vi "MES_Get StationData.vi"(0 "LineNum":string, 5 "StationName":string, 11 "error in (no error)":errorcluster, 12 "Alarm":bool=TRUE) -> (4 "Value":T1, 10 "Total Results":string[][](table), 13 "Table Control":string[][](array[string]), 14 "PLC DB DBB1List":string[](array[string]), 15 "error out":errorcluster)   [LabVIEW 2017, in "SQLite.lvclass"]
doc: "获取工位的使用的DB，结果DB，交互信号DB，报警DB，设备状态-结果分类-Andon报警DB、\n#2020-5-23 10:10:02\n蒋松\njiangsong@outlook.com"
uses:
  SQLite.lvclass
  Control/Station value Type.ctl
  SQLiteFileName.ctl
  TabelFullName.ctl
  <userlib>/LabSQL/LabSQL.lvlib
  <userlib>/sushu/sushu.lvlib
panel:
  in  "String":string
  out "number (0 to 1)":dbl
  out "Select SQL CMD":string
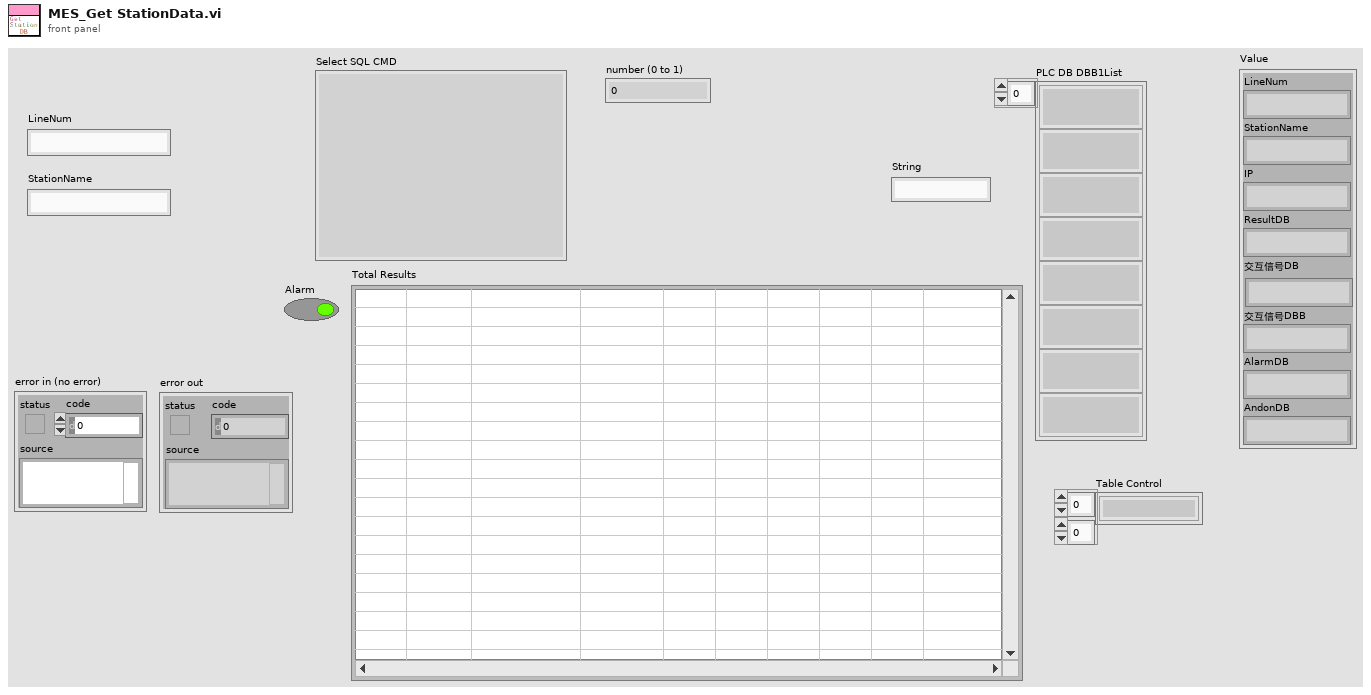
[diagram p1: front panel]
types:
  T1 = typedef "SQLite.lvclass/Station value Type.ctl" = cluster{"LineNum":string, "StationName":string, "IP":string, "ResultDB":string, "交互信号DB":string, "交互信号DBB":string, "AlarmDB":string, "AndonDB":string}
  T2 = enum16{"Initialize", "Read", "Write", "UnInitialize"}
  T3 = typedef "SQLite.lvclass/TabelFullName.ctl" = string
  T4 = typedef "SQLite.lvclass/SQLiteFileName.ctl" = string
  T5 = cluster{"Current VI Reference":refnum<vi>, "Close Panel on Exit?":bool}
  T6 = cluster{"Core":cluster{"Current VI Reference":refnum<vi>, "Close Panel on Exit?":bool}, "VI Name":string}
  T7 = enum16{"Other", "SQL2008", "SQLite", "Access", "MySQL"}
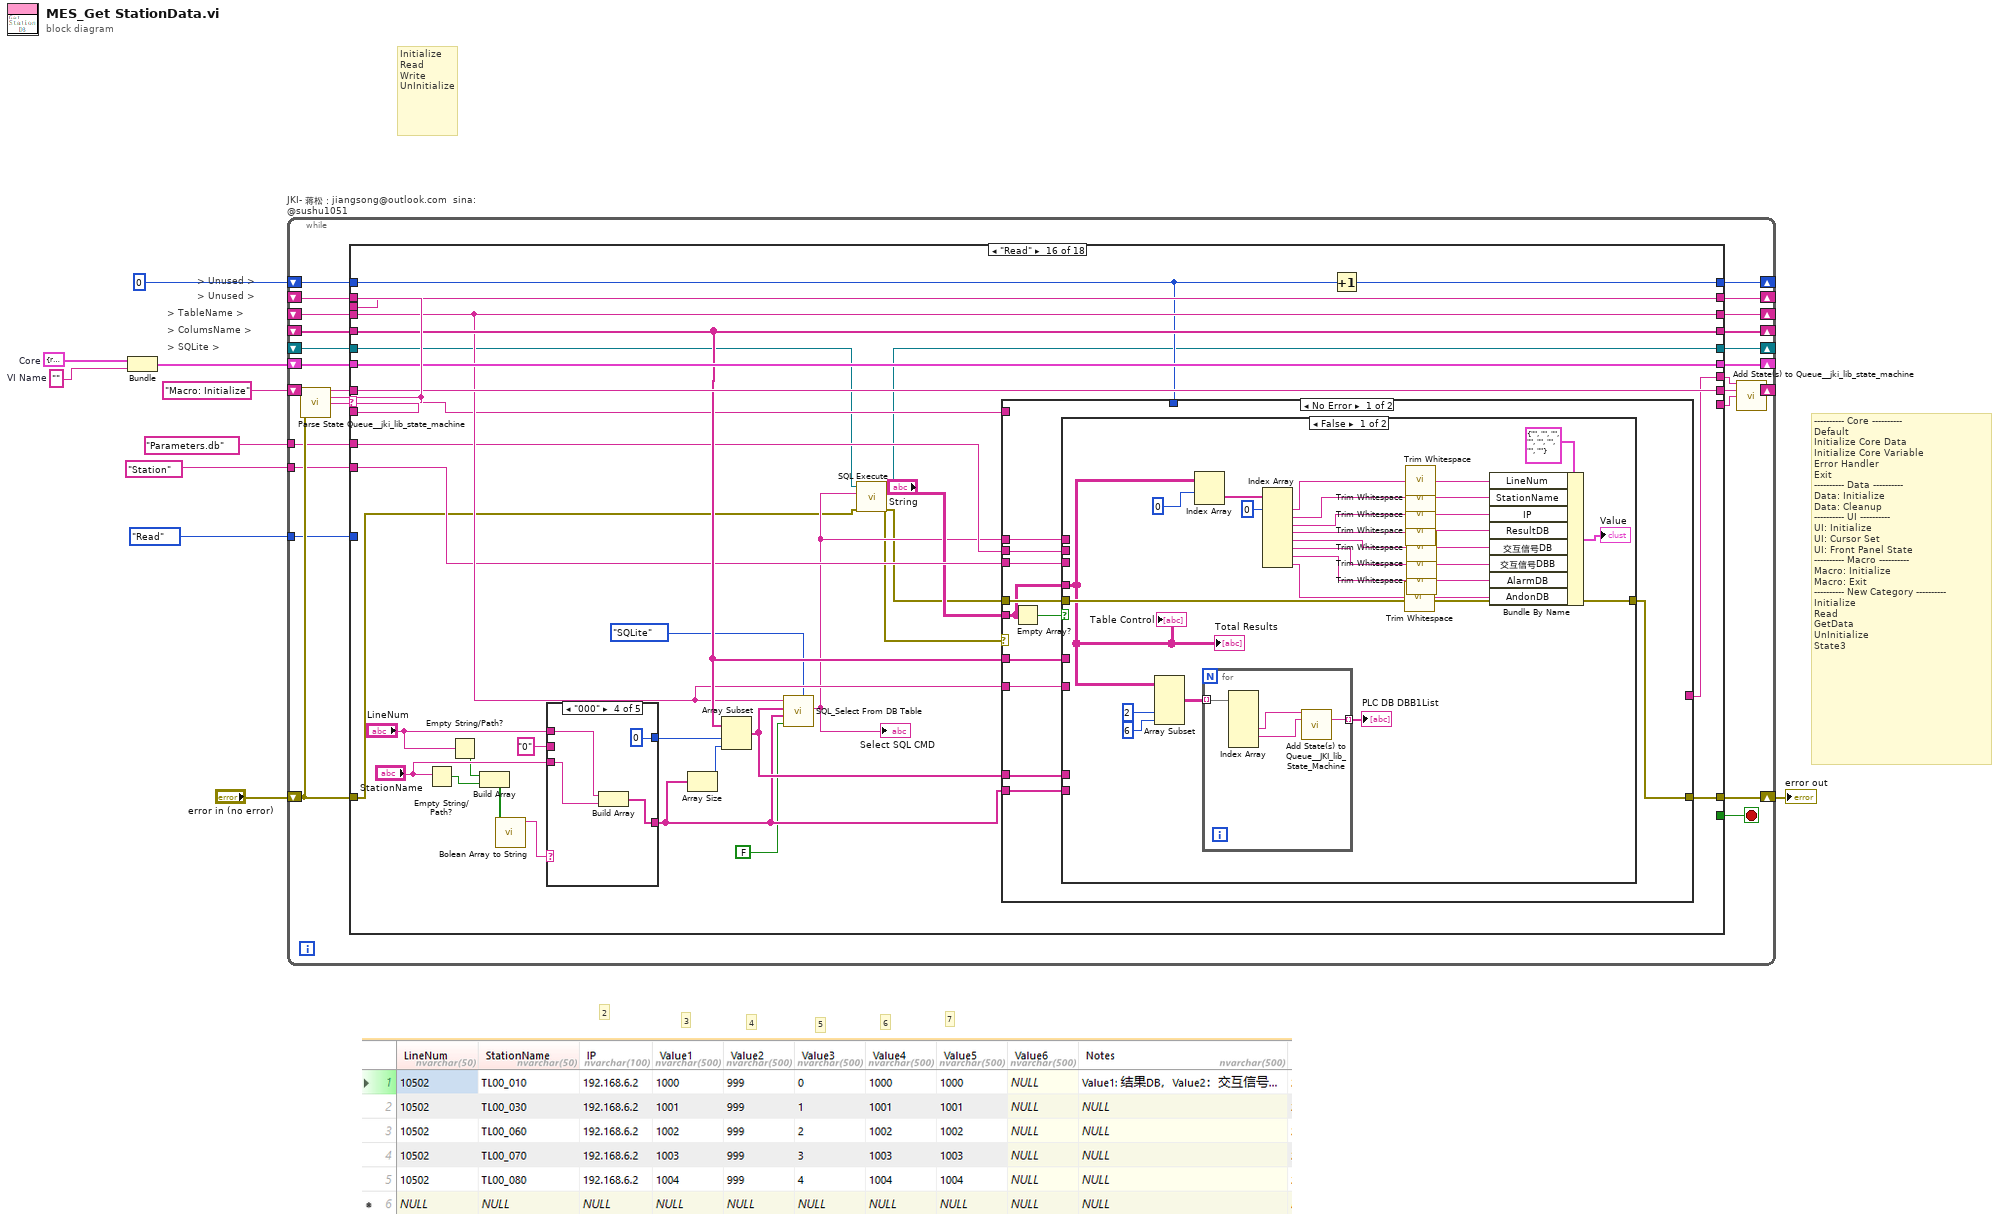
[diagram p0: block diagram]
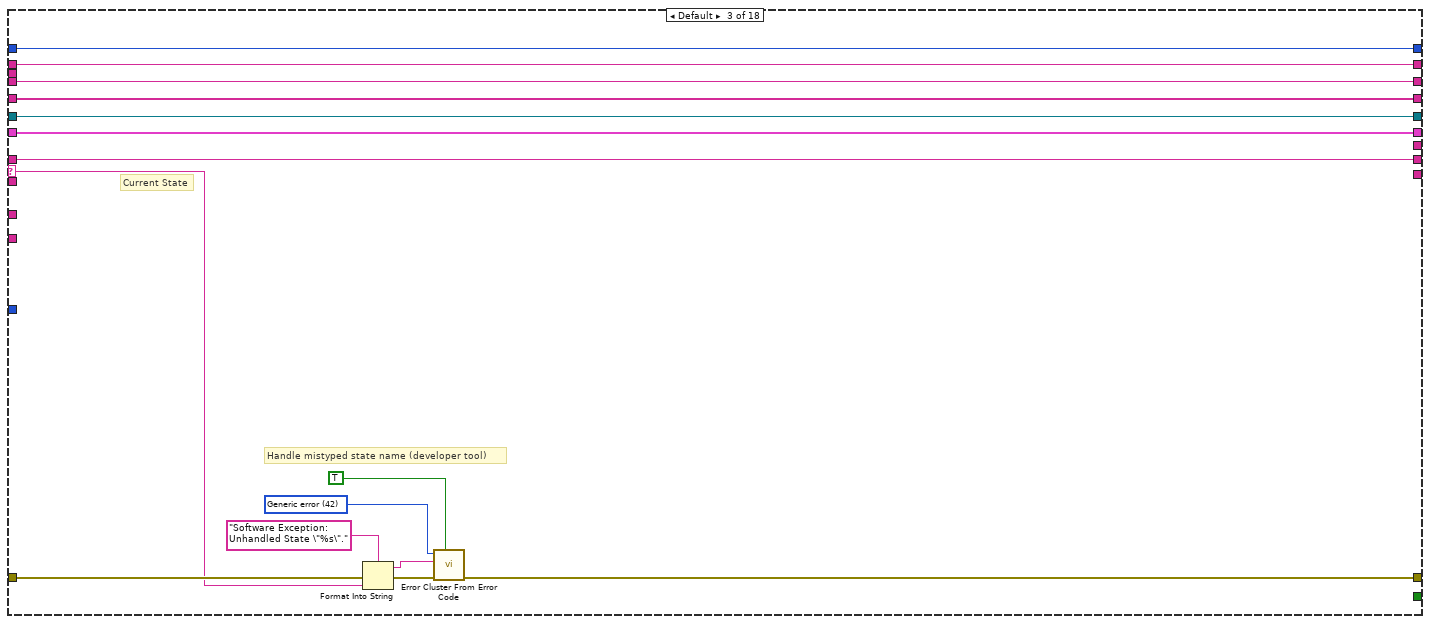
[diagram p4: hidden frame]
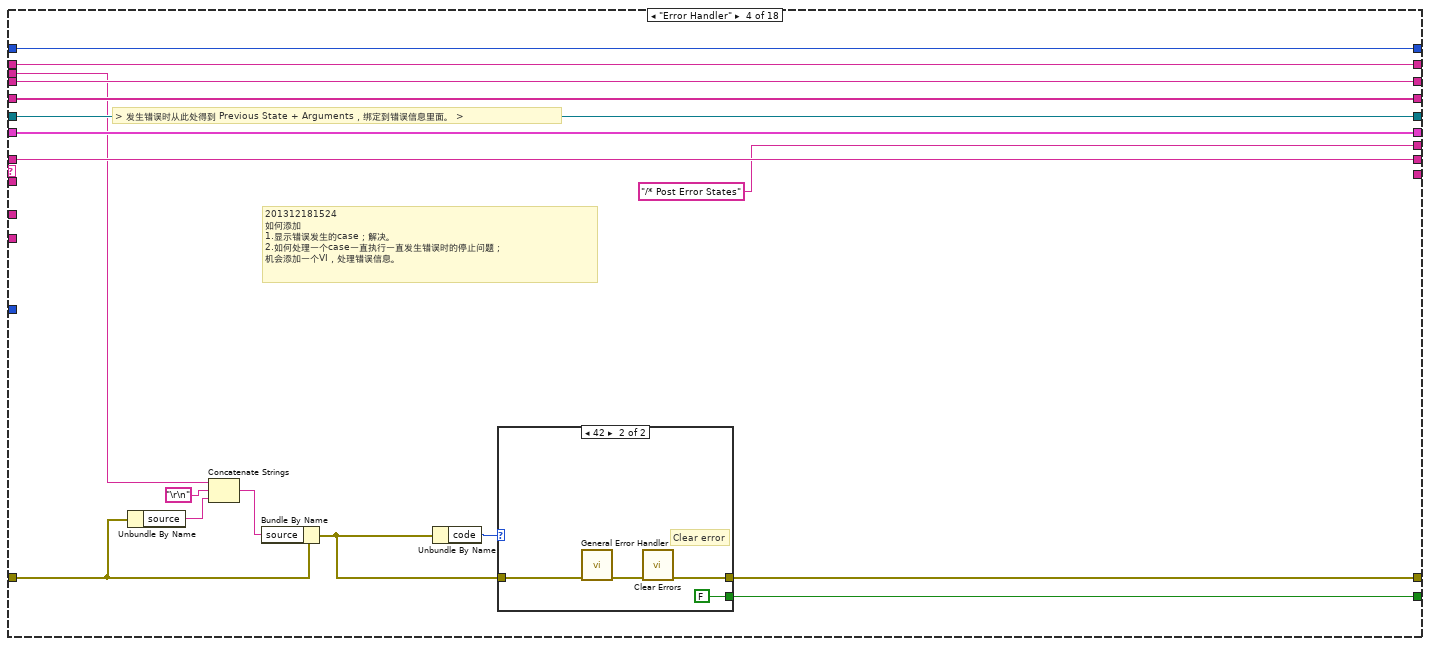
[diagram p5: hidden frame]
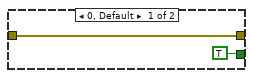
[diagram p6: hidden frame]
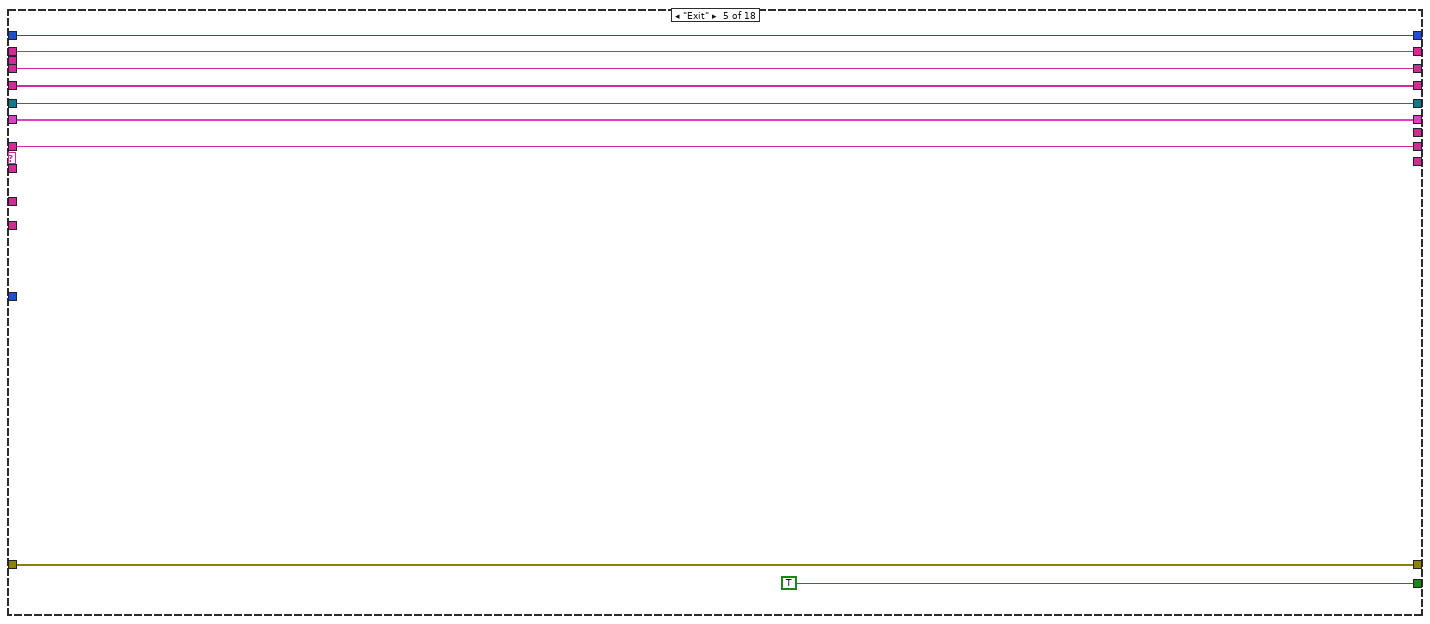
[diagram p7: hidden frame]
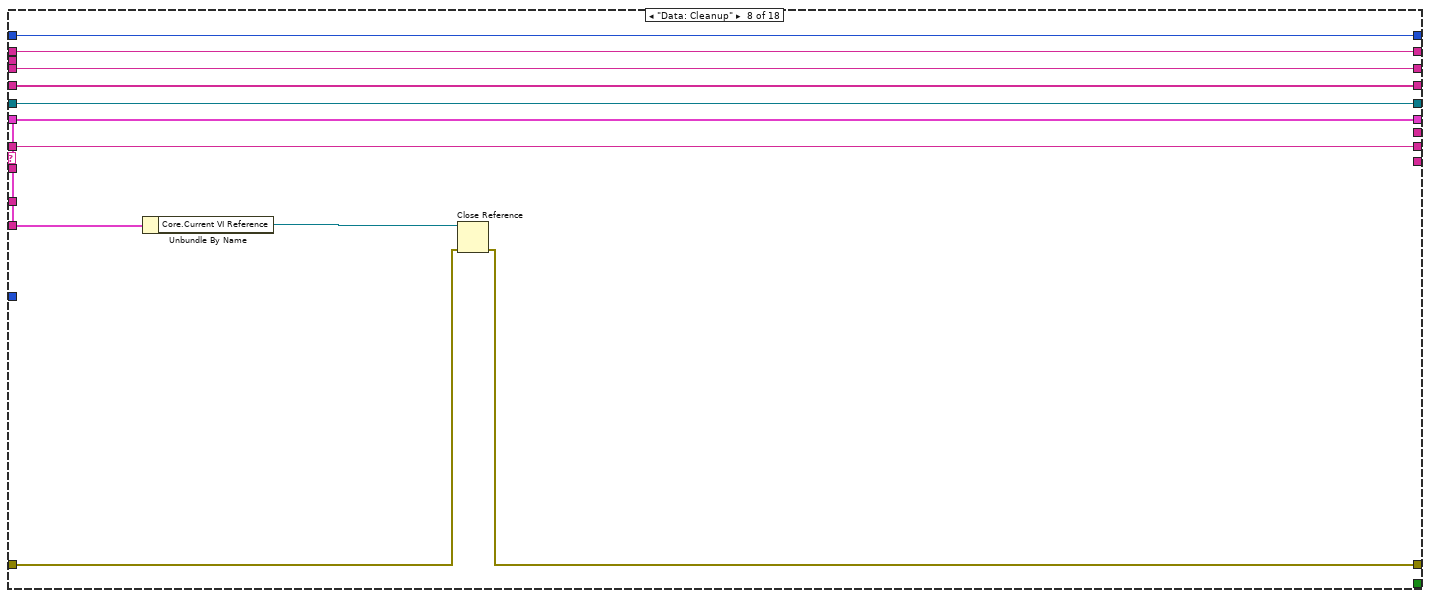
[diagram p10: hidden frame]
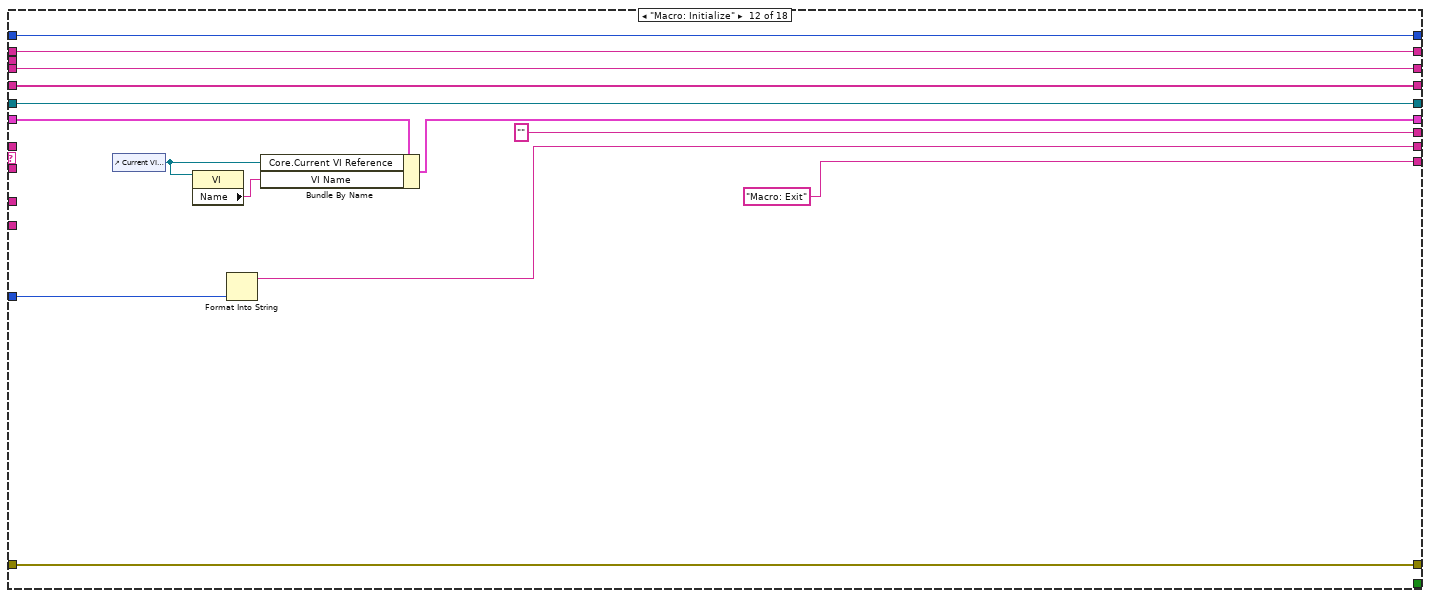
[diagram p14: hidden frame]
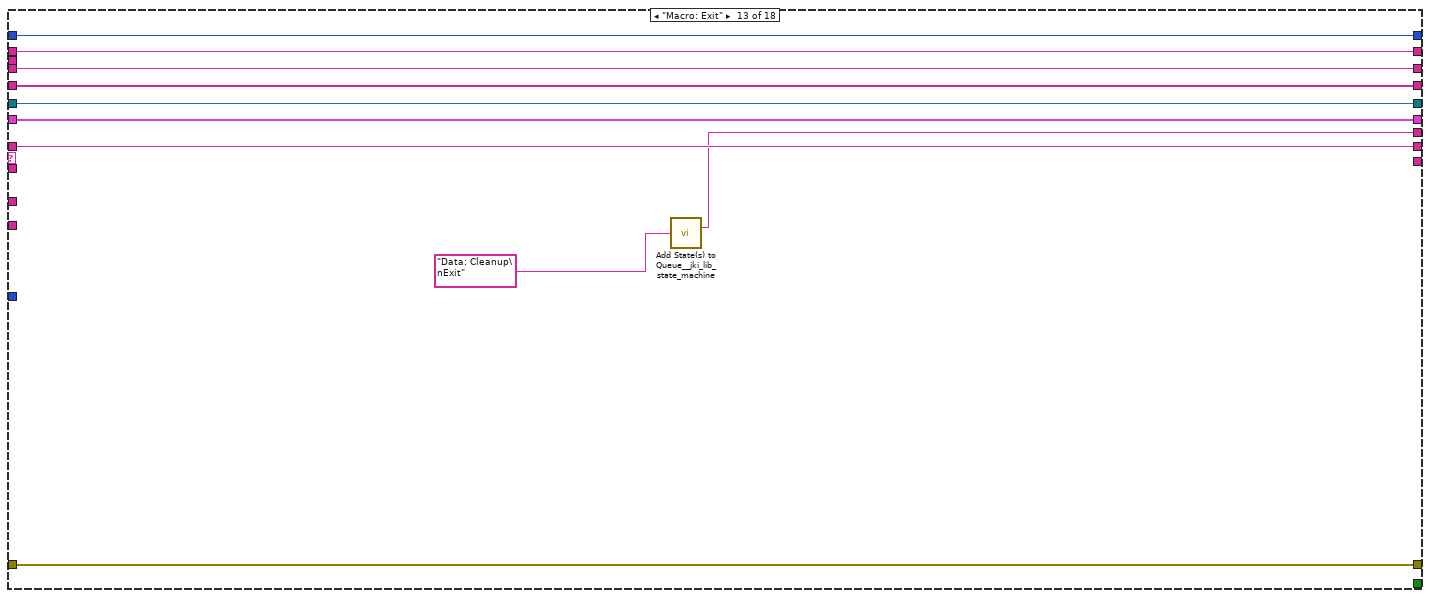
[diagram p15: hidden frame]
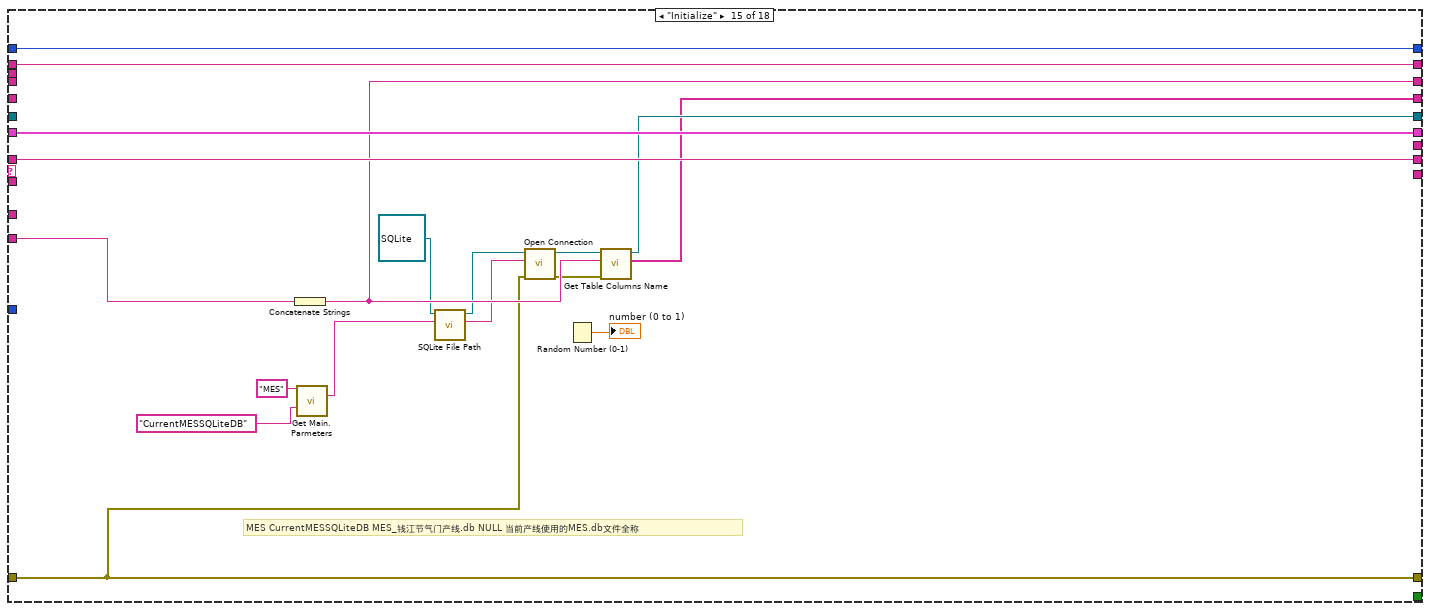
[diagram p17: hidden frame]
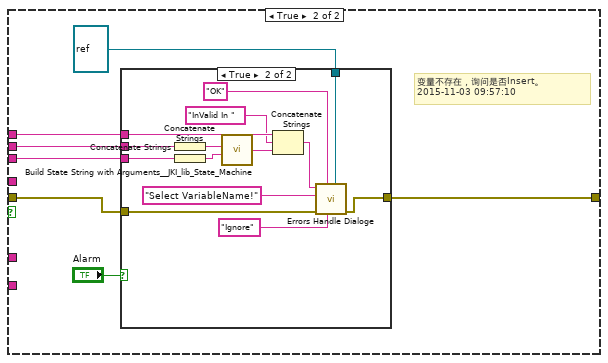
[diagram p18: hidden frame]
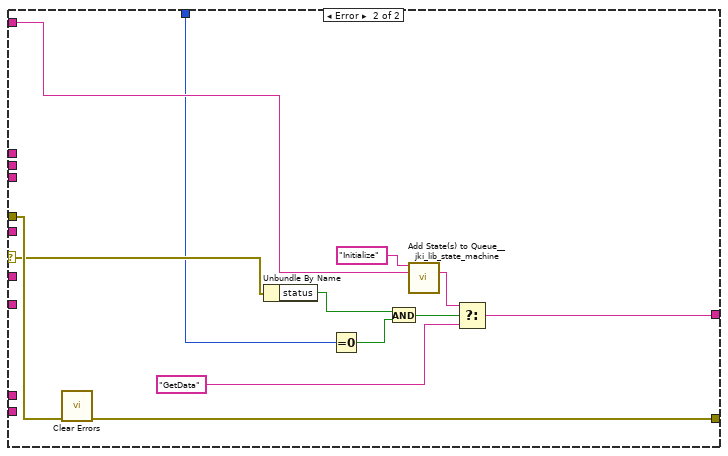
[diagram p20: hidden frame]
diagram:
  w10 = ""  # VI Name
  w9 = T5 {"Current VI Reference"=refnum, "Close Panel on Exit?"=FALSE}  # Core
  # "7"
  # "2"
  # "6"
  # "5"
  # "4"
  # "3"
  # "Initialize\nRead\nWrite\nUnInitialize"
  # "> Unused >"
  # "> SQLite >"
  # "> ColumsName >"
  # "> TableName >"
  # "> Unused >"
  # "---------- Core ----------\nDefault\nInitialize Core Data\nInitialize Core Variable\nError Handler\nExit\n---------- Data ----------\nData: Initialize\nData: Cleanup\n---------- UI ----------\nUI: Initialize\nUI: Cursor Set\nUI: Front Panel State\n---------- Macro ----------\nMacro: Initialize\nMacro: Exit\n---------- New Category ----------\nInitialize\nRead\nGetData\nUnInitialize\nState3"
  n1 = Bundle("Core"=w9, "VI Name"=w10) -> (w8:T6)  [unwired: 1 in]
  n2 = while "JKI- 蒋松：jiangsong@outlook.com  sina: @sushu1051" {
    shift-right: [w34] -> w3
    shift-left: "error in (no error)" -> [w32]
    shift-right: [w22] -> _
    shift-left: "Macro: Initialize" -> [w23]
    shift-right: [w29] -> _
    shift-left: _ -> [w31]
    shift-right: [w30] -> _
    shift-left: _ -> [w11]
    shift-right: [w24] -> _
    shift-left: w8 -> [w27]
    shift-right: [w25] -> _
    shift-left: _ -> [w18]
    shift-right: [w26] -> _
    shift-left: _ -> [w28]
    shift-right: [w17] -> _
    shift-left: 0 -> [w16]
    tunnel: T2."Read" ("CMD") -> [w15]
    tunnel: T4 "Parameters.db" ("SQLiteFileName") -> [w14]
    tunnel: T3 "Station" ("TabelFullName") -> [w13]
    stop <- w33 stop-if-true
    n3 = call <vilib>:"Parse State Queue__jki_lib_state_machine.vi"("State Queue"=w23, "Error In (no error)"=w32) -> ("Remaining States"=w36:string, "Current State"=w12:string, "Arguments"=w35:string)  [unwired: 10 in, 1 out]
    n4 = case shown="\"Read\"" w12 {
      selector: w12 -> [_ _ w55 _ _ _ _ _ _ _ _ _ _ _ _ w217 _ _]
      tunnel: w36 -> [w44 w46 w54 w76 w92 w101 w110 w117 w127 w135 w143 _ w166 w175 w199 w230 w331 w341]
      tunnel: w35 -> [_ _ _ _ _ _ _ _ _ _ _ _ _ _ _ _ _ _]
      tunnel: [w43 w52 w56 w70 w94 w103 w112 w119 w129 w137 w145 w160 w170 w178 w189 w218 w324 w332] -> w34
      tunnel: w32 -> [w43 w52 w57 w80 w94 w103 w112 w120 w129 w137 w145 w160 w170 w178 w189 w210 w324 w333]
      tunnel: [w44 w46 w54 w76 w92 w101 w110 w117 w127 w135 w143 w151 w166 w175 w199 w230 w331 w341] -> w21
      tunnel: [_ _ _ w69 TRUE _ _ _ _ _ _ _ _ _ _ _ _ _] -> w33
      tunnel: w12 -> [w42 w51 w67 w84 w99 w107 w115 w125 w133 w141 w149 w163 w173 w181 w198 w219 w325 w340]
      tunnel: w31 -> [w41 w50 w66 w83 w98 w106 w114 w124 w132 w140 w148 w162 w172 w180 _ w222 w330 w339]
      tunnel: [w42 w51 w67 w84 w99 w107 w115 w125 w133 w141 w149 w163 w173 w181 w198 w219 w325 w340] -> w30
      tunnel: [w41 w50 w66 w83 w98 w106 w114 w124 w132 w140 w148 w162 w172 w180 w191 w222 w330 w339] -> w29
      tunnel: w28 -> [w40 w49 w65 w82 w97 w105 w113 w123 w131 w139 w147 w161 w171 w179 _ w223 w329 w338]
      tunnel: w18 -> [w38 w47 w64 w74 w93 w102 w111 w118 w128 w136 w144 w159 w167 w176 _ w214 w328 w335]
      tunnel: w27 -> [w39 w48 w63 w81 w96 w104 w108 w121 w130 w138 w146 w153 w168 w177 w197 w229 w327 w337]
      tunnel: [w40 w49 w65 w82 w97 w105 w113 w123 w131 w139 w147 w161 w171 w179 w192 w223 w329 w338] -> w26
      tunnel: [w38 w47 w64 w74 w93 w102 w111 w118 w128 w136 w144 w159 w167 w176 w193 w212 w328 w334] -> w25
      tunnel: [w39 w48 w63 w81 w96 w104 w108 w121 w130 w138 w146 w152 w168 w177 w197 w229 w327 w337] -> w24
      tunnel: [_ _ _ "/* Post Error States" _ _ _ _ _ _ _ "" w165 _ _ w216 _ _] -> w20
      tunnel: [_ _ _ _ _ _ _ _ _ _ _ "Macro: Exit" _ _ _ _ _ _] -> w19
      tunnel: w16 -> [w37 w45 w53 w73 w91 w100 w109 w116 w126 w134 w142 w158 w164 w174 w196 w215 w326 w336]
      tunnel: [w37 w45 w53 w73 w91 w100 w109 w116 w126 w134 w142 w158 w164 w174 w196 w228 w326 w336] -> w17
      tunnel: w15 -> [_ _ _ _ _ _ _ _ _ _ _ w150 _ _ _ _ _ _]
      tunnel: w14 -> [_ _ _ _ _ _ _ _ _ _ _ _ _ _ _ w220 _ _]
      tunnel: w13 -> [_ _ _ _ _ _ _ _ _ _ _ _ _ _ w194 w221 _ _]
      tunnel: w11 -> [_ _ _ w68 _ _ _ _ _ _ _ _ _ _ _ _ _ _]
      frame "Idle" {
      }
      frame "---------- Core ----------" {
      }
      frame Default {
        w59 = 42 items=["No error", "Argument error", "Memory is full", "Out of zone", "End of file", "File already open", "Generic file I/O error", "File not found", "File permission error", "Disk is full", "Duplicate path", "Too many files open", "System feature not enabled", "Resource file not found", "Cannot add resource", "Resource not found", "Image not found", "Image memory error", "Pen does not exist", "Config type invalid", "Config token not found", "Config parse error", "Config memory error", "Bad external code format", "Bad external code offset", "External code not present", "Null window", "Destroy window error", "Null menu", "Print aborted", "Bad print record", "Print driver error", "Windows error during printing", "Memory error during printing", "Print dialog error", "Generic print error", "Invalid device refnum", "Device not found", "Device parameter error", "Device unit error", "Cannot open device", "Device call aborted", "Generic error", "Cancelled by user", "Object ID too low", "Object ID too high", "Object not in heap", "Unknown heap", "Unknown object (invalid DefProc)", "Unknown object (DefProc not in table)", "Message out of range", "Invalid (null) method", "Unknown message", "Manager call not supported", "Bad address", "Network operation in progress", "Network operation timed out", "Connection is busy", "Network attribute not supported", "Network error", "Address in use", "System out of memory", "Connection aborted", "Connection refused", "Not connected", "Already connected", "Connection closed", "Initialization error (interapplication manager)", "Bad occurrence", "Wait on unbound occurrence handler", "Occurrence queue overflow", "Datalog type conflict", "Unused", "Unrecognized type (interapplication manager)", "Memory corrupt", "Failed to make temporary DLL", "Old CIN version", "Drag socket not found", "Failed to load drop-object", "Failed to register OLE object", "Failed to release OLE object", "Format specifier type mismatch", "Unknown format specifier", "Too few format specifiers", "Too many format specifiers", "Scan failed", "Newer CIN version", "Error converting to variant", "Runtime menu error", "Password tampered", "Variant attribute not found", "Incompatible variant data type", "Event data is not available", "Event Store is not present", "Occurrence is not found", "Event Queue is not created", "Event info is not available", "Refnum passed is NULL", "Error retrieving Class GUID", "Error retrieving CoClass GUID", "Error retrieving TypeLib GUID.", "Bad built application magic bytes.", "Specific driver is different from the specific driver associated with the Logical Name.", "There is no session opened to the class driver.", "Max Error", "MAX - Error with config objects", "MAX - Error loading configuration", "MAX - Group not supported"]
        # "Current State"
        # "Handle mistyped state name (developer tool)"
        n5 = Format Into String(format string="Software Exception: Unhandled State \"%s\"." ("message"), error in=w57, w55) -> (resulting string=w60:string, error out=w61:errorcluster)  [unwired: 1 in]
        n6 = call <vilib>:"Error Cluster From Error Code.vi"("show call chain? (False)"=TRUE, "error in (no error)"=w61, "error message (\"\")"=w60, "error code (0)"=w59) -> ("error out"=w56:errorcluster)  [unwired: 5 in]
      }
      frame "Error Handler" {
        # "> 发生错误时从此处得到 Previous State + Arguments，绑定到错误信息里面。 >"
        # "201312181524\n如何添加\n1.显示错误发生的case；解决。\n2.如何处理一个case一直执行一直发生错误时的停止问题；\n机会添加一个VI，处理错误信息。"
        # "Clear error"
        n7 = Unbundle By Name(w80) -> ("source"=w78:string)
        n8 = Concatenate Strings(w68, "\r\n", w78) -> (w77:string)
        n9 = Bundle By Name(cluster=w80, "source"=w77) -> (w71:errorcluster)
        n10 = Unbundle By Name(w71) -> ("code"=w72:i32)
        n11 = case shown="42" w72 {
          tunnel: [TRUE FALSE] -> w69
          tunnel: w71 -> [w86 w89]
          tunnel: [w86 w87] -> w70
          frame 0, Default {
          }
          frame 42 {
            n12 = call <vilib>:"General Error Handler.vi"("error in (no error)"=w89) -> ("error out"=w88:errorcluster)  [unwired: 10 in, 4 out]
            n13 = call <vilib>:"Clear Errors.vi"("error in (no error)"=w88) -> ("error out"=w87:errorcluster)  [unwired: 5 in, 1 out]
          }
        }
      }
      frame "Exit" {
      }
      frame "---------- Data ----------" {
      }
      frame "Data: Initialize" {
      }
      frame "Data: Cleanup" {
        n14 = Unbundle By Name(w121) -> ("Core.Current VI Reference"=w122:refnum<vi>)
        n15 = Close Reference(reference=w122, error in (no error)=w120) -> (error out=w119:errorcluster)
      }
      frame "---------- UI ----------" {
      }
      frame "UI: Initialize" {
      }
      frame "---------- Macro ----------" {
      }
      frame "Macro: Initialize" {
        n16 = control-ref of="Current VI Reference"() -> (w154:refnum<vi>)
        n17 = property class="VI"(reference=w154) -> ("Name"=w155:string)  [unwired: 1 in, 2 out]
        n18 = Format Into String(w150) -> (resulting string=w151:string)  [unwired: 3 in, 1 out]
        n19 = Bundle By Name(cluster=w153, "Core.Current VI Reference"=w154, "VI Name"=w155) -> (w152:T6)
      }
      frame "Macro: Exit" {
        n20 = call <vilib>:"Add State(s) to Queue__jki_lib_state_machine.vi"("State(s) at Back (\"\")"="Data: Cleanup\nExit") -> ("States Out"=w165:string)  [unwired: 14 in]
      }
      frame "---------- New Category ----------" {
      }
      frame "Initialize" {
        # "MES\tCurrentMESSQLiteDB\tMES_钱江节气门产线.db\tNULL\t当前产线使用的MES.db文件全称"
        n21 = Concatenate Strings(w194) -> (w191:string)
        n22 = call "Get Main.Parmeters.vi"("Main"="MES", "VariableName"="CurrentMESSQLiteDB" ("Main")) -> ("Value"=w182:string)  [unwired: 6 in, 7 out]
        n23 = call "SQLite File Path.vi"("SQLiteFileName"=w182, "SQLite in"=refnum<class "SQLite.lvclass"> refnum ("SQLite.lvclass")) -> ("string"=w188:string, "SQLite out"=w186:refnum<class "SQLite.lvclass">)  [unwired: 7 in, 1 out]
        n24 = call-dynamic "Open Connection.vi"("error in (no error)"=w189, "ConnectionString"=w188, "HostDB in"=w186) -> ("error out"=w190:errorcluster, "HostDB out"=w195:refnum<class "SQLite.lvclass">)  [unwired: 7 in]
        n25 = Random Number (0-1)() -> (number: 0 to 1=→"number (0 to 1)":dbl)
        n26 = call-dynamic "Get Table Columns Name.vi"("error in (no error)"=w190, "TableName"=w191, "HostDB in"=w195) -> ("Table_ColunmsList"=w192:string[], "HostDB out"=w193:refnum<class "SQLite.lvclass">)  [unwired: 4 in, 3 out]
      }
      frame "Read" {
        n27 = Empty String/Path?(string/path="StationName") -> (empty?=w207:bool)
        n28 = Empty String/Path?(string/path="LineNum") -> (empty?=w202:bool)
        n29 = Build Array(w202, w207) -> (w206:bool[])
        n30 = call <userlib>:"Bolean Array to String.vi"("Bolean Array"=w206) -> ("Bolean String"=w205:string)  [unwired: 10 in]
        n31 = case shown="\"000\"" w205 {
          tunnel: [w309 w312 w315 w319 w323] -> w226
          tunnel: "StationName" -> [w307 _ _ w316 w322]
          tunnel: [1 ("index") 2 ("index") 0 ("index") 0 ("index") 0 ("index")] -> w203
          tunnel: "LineNum" -> [_ _ w313 w317 w320]
          tunnel: "0" ("element") -> [_ _ _ _ _]
          frame "10" {
            n32 = Build Array(w307) -> (w309:string[])
          }
          frame "11" {
            n33 = Build Array("" ("element")) -> (w312:string[])
          }
          frame "01" {
            n34 = Build Array(w313) -> (w315:string[])
          }
          frame "000" {
            n35 = Build Array(w317, w316) -> (w319:string[])
          }
          frame "False", Default {
            n36 = Build Array(w320, w322) -> (w323:string[])
          }
        }
        n37 = Array Size(array=w226) -> (size(s)=w225:i32)
        n38 = Array Subset(array=w223, index=w203, length=w225) -> (w227:string[])
        n39 = call <userlib>:"SQL_Select From DB Table.vi"("DB Type"=T7."SQLite", "Check ASCII?"=FALSE, "ColumnsValue"=w226, "ColumnsNameList"=w227, "TableName"=w222) -> ("Select SQL CMD"=w211:string)  [unwired: 6 in]
        "Select SQL CMD" <- w211
        n40 = call-dynamic "SQL Execute.vi"("error in (no error)"=w210, "Command Text"=w211, "HostDB in"=w214) -> ("error out"=w209:errorcluster, "Table Control"=w213:string[][], "HostDB out"=w212:refnum<class "SQLite.lvclass">)  [unwired: 4 in, 2 out]
        n41 = case shown="No Error" w209 {
          selector: w209 -> [_ w299]
          tunnel: w227 -> [w241 _]
          tunnel: w209 -> [w240 w306]
          tunnel: w211 -> [w238 _]
          tunnel: w213 -> [w237 _]
          tunnel: w226 -> [w236 _]
          tunnel: w223 -> [w235 _]
          tunnel: w222 -> [w234 _]
          tunnel: w221 -> [w233 _]
          tunnel: w220 -> [w232 _]
          tunnel: [w231 w305] -> w218
          tunnel: w217 -> [_ w298]
          tunnel: [_ w297] -> w216
          tunnel: w215 -> [_ w296]
          frame No Error {
            n42 = Empty Array?(array=w237) -> (empty?=w239:bool)
            n43 = case shown="False" w239 {
              tunnel: [w268 w278] -> w231
              tunnel: w235 -> [_ _]
              tunnel: w234 -> [_ _]
              tunnel: w236 -> [_ _]
              tunnel: w241 -> [_ _]
              tunnel: w240 -> [w268 w279]
              tunnel: w238 -> [_ w275]
              tunnel: w232 -> [_ w277]
              tunnel: w233 -> [_ w276]
              tunnel: w237 -> [w254 _]
              frame False {
                n44 = Array Subset(array=w254, index (col)=2 ("index"), length (col)=6 ("length")) -> (w259:string[][])  [unwired: 2 in]
                n45 = Index Array(array=w254, index (row)=0) -> (element=w266:string[])  [unwired: 1 in]
                n46 = for {
                  tunnel: w259 -> [w272] mode=indexing
                  tunnel: [w271] -> w258 mode=indexing
                  n47 = Index Array(array=w272) -> (element #3=w270:string, element #4=w269:string)  [unwired: 5 in, 3 out]
                  n48 = call <vilib>:"Add State(s) to Queue__JKI_lib_State_Machine.vi"("State(s) in Front (\"\")"=w270, "State(s) in (\"\")"=w269) -> ("States Out"=w271:string)  [unwired: 13 in]
                }
                "PLC DB DBB1List" <- w258
                n49 = Index Array(array=w266, index #1=0 ("index")) -> (element #1=w265:string, element #2=w264:string, element #3=w263:string, element #4=w262:string, element #5=w247:string, element #6=w246:string, element #7=w245:string, element #8=w244:string)  [unwired: 7 in]
                n50 = call <vilib>:"Trim Whitespace.vi"("string"=w244) -> ("trimmed string"=w243:string)  [unwired: 1 in]
                n51 = call <vilib>:"Trim Whitespace.vi"("string"=w265) -> ("trimmed string"=w257:string)  [unwired: 1 in]
                n52 = call <vilib>:"Trim Whitespace.vi"("string"=w264) -> ("trimmed string"=w256:string)  [unwired: 1 in]
                n53 = call <vilib>:"Trim Whitespace.vi"("string"=w263) -> ("trimmed string"=w255:string)  [unwired: 1 in]
                n54 = call <vilib>:"Trim Whitespace.vi"("string"=w262) -> ("trimmed string"=w250:string)  [unwired: 1 in]
                n55 = call <vilib>:"Trim Whitespace.vi"("string"=w247) -> ("trimmed string"=w249:string)  [unwired: 1 in]
                n56 = call <vilib>:"Trim Whitespace.vi"("string"=w246) -> ("trimmed string"=w248:string)  [unwired: 1 in]
                n57 = call <vilib>:"Trim Whitespace.vi"("string"=w245) -> ("trimmed string"=w242:string)  [unwired: 1 in]
                n58 = Bundle By Name(cluster=T1 {"LineNum"="", "StationName"="", "IP"="", "ResultDB"="", "交互信号DB"="", "交互信号DBB"="", "AlarmDB"="", "AndonDB"=""} ("Value"), "LineNum"=w257, "StationName"=w256, "IP"=w255, "ResultDB"=w250, "交互信号DB"=w249, "交互信号DBB"=w248, "AlarmDB"=w242, "AndonDB"=w243) -> (→"Value":T1)
                "Total Results" <- w254
                "Table Control" <- w254
              }
              frame True {
                # "变量不存在，询问是否Insert。\n2015-11-03 09:57:10"
                n59 = case shown="True" "Alarm" {
                  tunnel: w279 -> [w280 w294]
                  tunnel: [w280 w293] -> w278
                  tunnel: w277 -> [_ w292]
                  tunnel: w276 -> [_ w291]
                  tunnel: w275 -> [_ w290]
                  tunnel: refnum<vi> refnum ("VI Ref") -> [_ w281]
                  frame False {
                  }
                  frame True {
                    n60 = Concatenate Strings(w292) -> (w289:string)
                    n61 = Concatenate Strings(w291) -> (w288:string)
                    n62 = call <vilib>:"Build State String with Arguments__JKI_lib_State_Machine.vi"("Arguments (\"\")"=w288, "State"=w289) -> ("State with Arguments"=w286:string)  [unwired: 4 in]
                    n63 = Concatenate Strings(w290, "InValid In " ("Message"), w286) -> (w285:string)
                    n64 = call <userlib>:"Errors Handle Dialoge.vi"("VI Ref"=w281, "Cancel Text"="Ignore", "OK Text"="OK", "error in (no error)"=w294, "Title Text"="Select VariableName!", "Message"=w285) -> ("error out"=w293:errorcluster)  [unwired: 4 in, 1 out]
                  }
                }
              }
            }
          }
          frame Error {
            n65 = call <vilib>:"Clear Errors.vi"("error in (no error)"=w306) -> ("error out"=w305:errorcluster)  [unwired: 5 in, 1 out]
            n66 = Unbundle By Name(w299) -> ("status"=w295:bool)
            n67 = Equal To 0?(x=w296) -> (x = 0?=w303:bool)
            n68 = And(x=w295, y=w303) -> (x .and. y?=w302:bool)
            n69 = call <vilib>:"Add State(s) to Queue__jki_lib_state_machine.vi"("State(s) in Front (\"\")"="Initialize" ("Remaining States"), "State(s) in (\"\")"=w298) -> ("States Out"=w300:string)  [unwired: 13 in]
            n70 = Select(t=w300, s=w302, f="GetData") -> (s? t:f=w297:string)
          }
        }
        n71 = Increment(x=w215) -> (x+1=w228:i32)
      }
      frame "GetData" {
      }
      frame "UnInitialize" {
        n72 = call-dynamic "Close Connection.vi"("error in (no error)"=w333, "HostDB in"=w335) -> ("error out"=w332:errorcluster, "HostDB out"=w334:refnum<class "SQLite.lvclass">)  [unwired: 8 in]
      }
    }
    n73 = call <vilib>:"Add State(s) to Queue__jki_lib_state_machine.vi"("State(s) in Front (\"\")"=w20, "State(s) in (\"\")"=w21, "State(s) at Back (\"\")"=w19) -> ("States Out"=w22:string)  [unwired: 12 in]
  }
  "error out" <- w3
